vi "CreateSQLstring.vi"(10 "Table":string, 11 "Groups":string[](array[string])) -> (3 "SQL String":string)   [LabVIEW 2017, in "Server.lvlib" / "Oracle.lvlib"]
doc: "Creates the SQL String for the Oracle Database Query."
uses:
  Oracle.lvlib
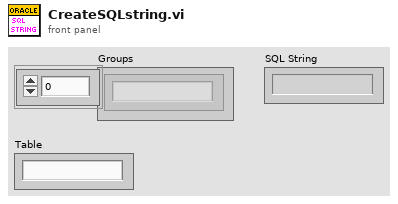
[diagram p1: front panel]
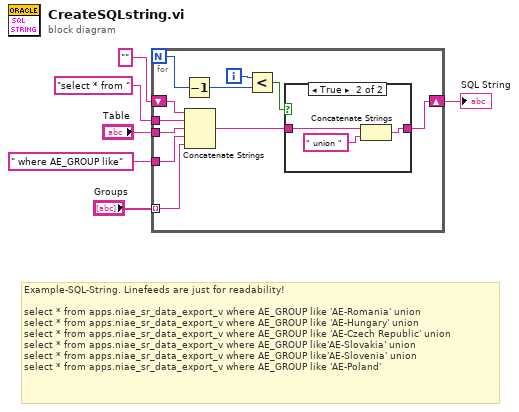
[diagram p0: block diagram]
diagram:
  # "Example-SQL-String. Linefeeds are just for readability!\n\nselect * from apps.niae_sr_data_export_v where AE_GROUP like 'AE-Romania' union \nselect * from apps.niae_sr_data_export_v where AE_GROUP like 'AE-Hungary' union \nselect * from apps.niae_sr_data_export_v where AE_GROUP like 'AE-Czech Republic' union \nselect * from apps.niae_sr_data_export_v where AE_GROUP like'AE-Slovakia' union \nselect * from apps.niae_sr_data_export_v where AE_GROUP like'AE-Slovenia' union \nselect * from apps.niae_sr_data_export_v where AE_GROUP like 'AE-Poland'"
  n1 = for {
    N -> [w17]
    tunnel: "Groups" -> [w9] mode=indexing
    shift-right: [w12] -> w6
    shift-left: "" -> [w11]
    tunnel: "Table" -> [w10]
    tunnel: " where AE_GROUP like" ("string") -> [w8]
    tunnel: "select * from " ("SQL query") -> [w7]
    i -> [w16]
    n2 = Decrement(x=w17) -> (x-1=w15:i32)
    n3 = Concatenate Strings(w11, w7, w10, w8, w9) -> (w13:string)
    n4 = Less?(x=w16, y=w15) -> (x < y?=w14:bool)
    n5 = case shown="True" w14 {
      tunnel: w13 -> [w18 w21]
      tunnel: [w18 w19] -> w12
      frame False {
      }
      frame True {
        n6 = Concatenate Strings(w21, " union " ("string")) -> (w19:string)
      }
    }
  }
  "SQL String" <- w6
